vi "InitializeRingTimeADC.vi"(8 "error in (no error)":errorcluster) -> (0 "error out":errorcluster, 3 "Ring Time ADC Task":refnum<k21>)   [LabVIEW 2019, in "Initialize.lvlib"]
uses:
  Initialize.lvlib
  <vilib>/DAQmx/create/channels.llb/DAQmx Create Channel (AI-Voltage-Basic).vi
  <vilib>/DAQmx/configure/timing.llb/DAQmx Timing (Sample Clock).vi
  <vilib>/DAQmx/configure/trigger.llb/DAQmx Start Trigger (Digital Edge).vi
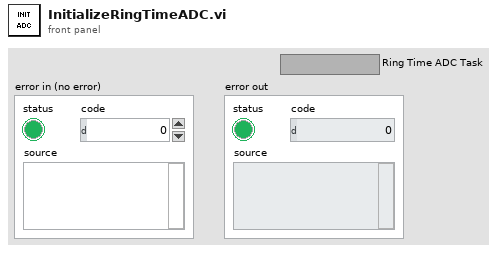
[diagram p1: front panel]
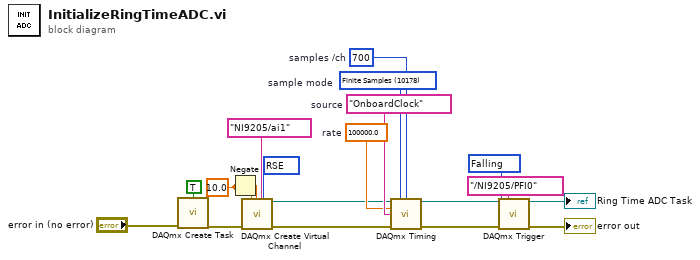
[diagram p0: block diagram]
diagram:
  w19 = 10.0 ("minimum value")
  w14 = tag "OnboardClock"  # source
  w11 = 100000.0  # rate
  w9 = 10171 items=["Rising"=10280, "Falling"=10171] ("slope")
  w8 = 700  # samples /ch
  w3 = 10178 items=["Finite Samples"=10178, "Continuous Samples"=10123, "Hardware Timed Single Point"=12522]  # sample mode
  w2 = 10083 items=["Default"=-1, "RSE"=10083, "NRSE"=10078, "Differential"=10106, "Pseudodifferential"=12529] ("input terminal configuration")
  n1 = call <vilib>:"DAQmx Create Task.vi"("auto cleanup"=TRUE, "error in"="error in (no error)") -> ("error out"=w16:errorcluster)  [unwired: 12 in, 1 out]
  n2 = Negate(x=w19) -> (-x=w18:dbl)
  n3 = call-poly <vilib>:"DAQmx Create Virtual Channel.vi"("maximum value"=w19, "minimum value"=w18, "input terminal configuration"=w2, "physical channels"=tag "NI9205/ai1", "error in"=w16) -> ("task out"=w6:refnum<k21>, "error out"=w7:errorcluster)  [unwired: 9 in]
  n4 = call-poly <vilib>:"DAQmx Timing.vi"("task/channels in"=w6, "sample mode"=w3, "samples per channel"=w8, "rate"=w11, "source"=w14, "error in"=w7) -> ("task out"=w4:refnum<k21>, "error out"=w5:errorcluster)  [unwired: 8 in]
  n5 = call-poly <vilib>:"DAQmx Trigger.vi"("task/channels in"=w4, "source"=tag "/NI9205/PFI0", "edge"=w9, "error in"=w5) -> ("task out"=→"Ring Time ADC Task":refnum<k21>, "error out"=→"error out":errorcluster)  [unwired: 10 in]
